vi "启动.vi"() -> ()   [LabVIEW 2016]
uses:
  <vilib>/NI/Progress Bar/Controls/Update Bar Actions.ctl
  <vilib>/NI/Progress Bar/Controls/Progress Bar Properties.ctl
  <vilib>/NI/Progress Bar/Progress Bar.lvlib
panel:
  out "exists?":bool
  out "error out":errorcluster
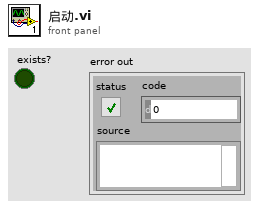
[diagram p1: front panel]
types:
  T1 = enum32{"Invalid", "Standard", "Closed", "Hidden", "Minimized", "Maximized"}
  T2 = typedef "Progress Bar.lvlib/Progress Bar Properties.ctl" = cluster{"Background Color":u32, "Installer Title":string, "Title Color":u32, "Action Text":string, "Text Color":u32, "Slider Value":u8, "Bar Color":u32, "Timeout":i32}
  T3 = typedef "Progress Bar.lvlib/Update Bar Actions.ctl" = enum16{"Add To Existing", "Set to Value"}
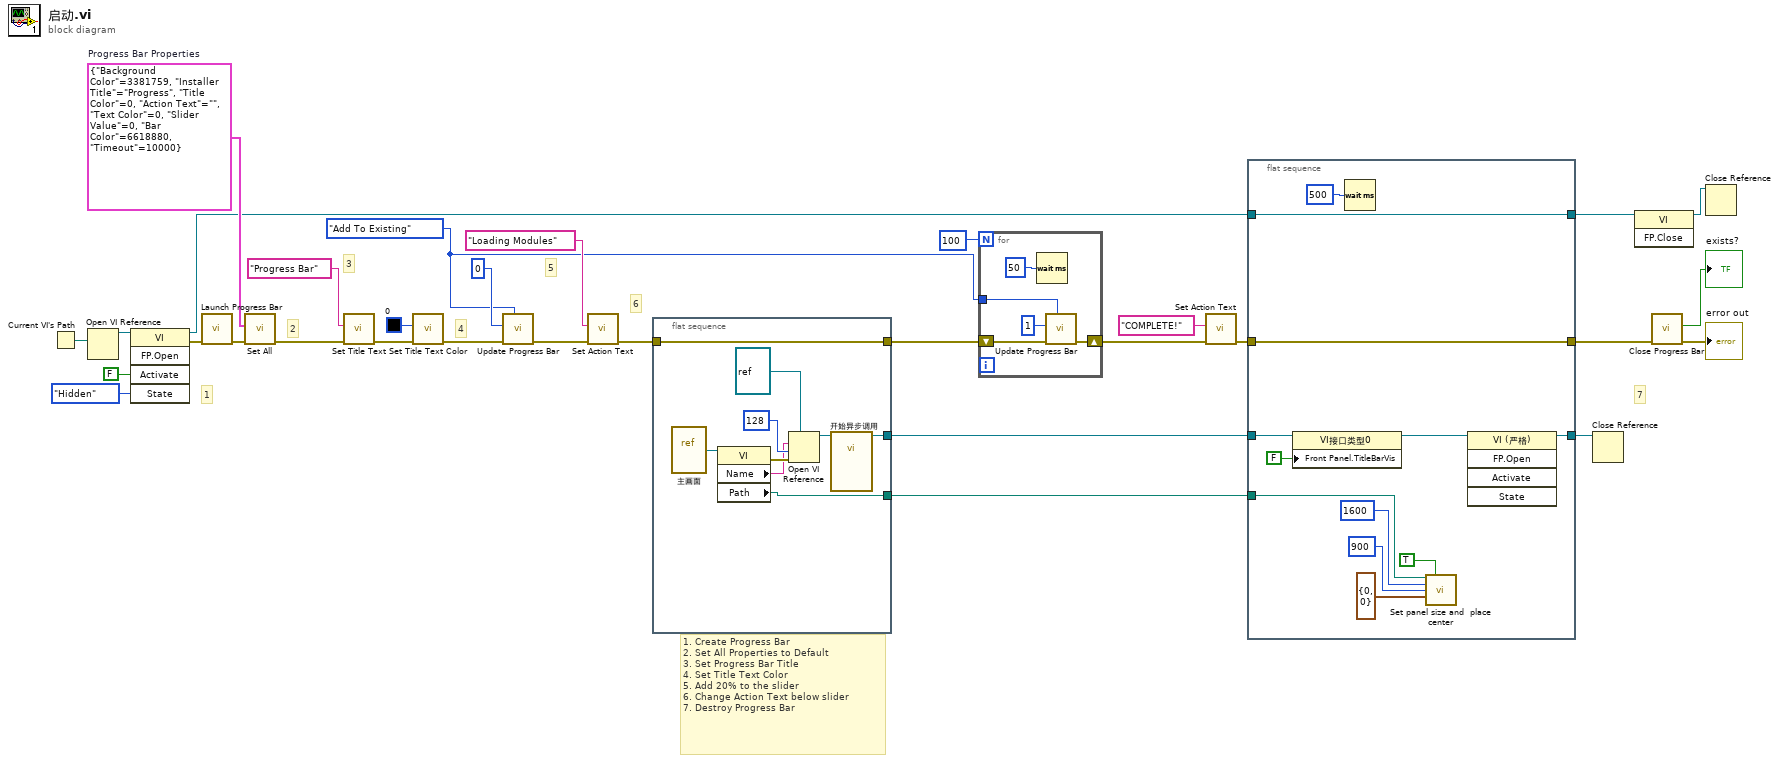
[diagram p0: block diagram]
diagram:
  w16 = T2 {"Background Color"=3381759, "Installer Title"="Progress", "Title Color"=0, "Action Text"="", "Text Color"=0, "Slider Value"=0, "Bar Color"=6618880, "Timeout"=10000}  # Progress Bar Properties
  w15 = Update_Bar_Actions."Add To Existing" ("Action")
  # "7"
  # "6"
  # "5"
  # "4"
  # "3"
  # "2"
  # "1"
  # "1. Create Progress Bar\n2. Set All Properties to Default\n3. Set Progress Bar Title\n4. Set Title Text Color\n5. Add 20% to the slider\n6. Change Action Text below slider\n7. Destroy Progress Bar"
  n1 = Current VI's Path() -> (path=w5:path)
  n2 = Open VI Reference(vi path=w5) -> (vi reference=w6:refnum<vi>)  [unwired: 5 in, 1 out]
  n3 = invoke class="VI" method="FP.Open"(reference=w6, "Activate"=FALSE ("激活？"), "State"=T1."Hidden" ("状态")) -> (reference out=w1:refnum<vi>, error out=w2:errorcluster)  [unwired: 2 in, 3 out]
  n4 = call <vilib>:"Launch Progress Bar.vi"("error in (no error)"=w2) -> ("error out"=w17:errorcluster)  [unwired: 9 in, 1 out]
  n5 = call <vilib>:"Set All.vi"("error in (no error)"=w17, "Progress Bar Properties (Default)"=w16) -> ("error out"=w27:errorcluster)  [unwired: 9 in]
  n6 = call <vilib>:"Set Title Text.vi"("error in (no error)"=w27, "Installer Title"="Progress Bar") -> ("error out"=w30:errorcluster)  [unwired: 9 in]
  n7 = call <vilib>:"Set Title Text Color.vi"("error in (no error)"=w30, "Color Box"=u32 0) -> ("error out"=w26:errorcluster)  [unwired: 9 in]
  n8 = call <vilib>:"Update Progress Bar.vi"("Action"=w15, "error in (no error)"=w26, "Value"=u8 0) -> ("error out"=w25:errorcluster)  [unwired: 8 in]
  n9 = call <vilib>:"Set Action Text.vi"("error in (no error)"=w25, "Action Text"="Loading Modules") -> ("error out"=w24:errorcluster)  [unwired: 9 in]
  n10 = flat-sequence {
    tunnel: w24 -> [w40]
    tunnel: [w40] -> w22
    tunnel: [w39] -> w9
    tunnel: [w32] -> w7
    frame #0 {
      n11 = vi-ref "主画面.vi"() -> (w34:refnum<vi>)
      n12 = property class="VI"(reference=w34) -> (error out=w38:errorcluster, "Name"=w35:string, "Path"=w32:path)  [unwired: 1 in, 1 out]
      n13 = Open VI Reference(type specifier VI Refnum (for type only)=refnum<vi> refnum ("类型说明符VI引用句柄（仅用于类型）"), vi path=w35, options=128 ("选项"), error in (no error)=w38) -> (vi reference=w33:refnum<vi>)  [unwired: 2 in, 1 out]
      n14 = call-by-ref "开始异步调用"(reference=w33) -> (reference out=w39:refnum<vi>)  [unwired: 13 in, 1 out]
    }
  }
  n15 = for {
    N: 100 ("Value") -> [_]
    tunnel: w15 -> [w42]
    shift-right: [w45] -> w21
    shift-left: w22 -> [w44]
    n16 = Wait (ms)(milliseconds to wait=u32 50) -> ()  [unwired: 1 out]
    n17 = call <vilib>:"Update Progress Bar.vi"("Action"=w42, "error in (no error)"=w44, "Value"=u8 1) -> ("error out"=w45:errorcluster)  [unwired: 8 in]
  }
  n18 = call <vilib>:"Set Action Text.vi"("error in (no error)"=w21, "Action Text"="COMPLETE!") -> ("error out"=w20:errorcluster)  [unwired: 9 in]
  n19 = flat-sequence {
    tunnel: w20 -> [w56]
    tunnel: [w56] -> w18
    tunnel: [w55] -> w10
    tunnel: w1 -> [w55]
    tunnel: w9 -> [w48]
    tunnel: [w54] -> w8
    tunnel: w7 -> [w49]
    frame #0 {
      n20 = property class="VI接口类型0"(reference=w48, "Front Panel.TitleBarVis"=FALSE ("前面板窗口:标题栏可见")) -> (reference out=w47:refnum<vi>)  [unwired: 1 in, 1 out]
      n21 = Wait (ms)(milliseconds to wait=u32 500) -> ()  [unwired: 1 out]
      n22 = call "Set panel size and  place center.vi"("Path"=w49, "Close Reference (false)"=TRUE, "Panel Width"=1600, "Panel Height"=900, "FP.Origin in(H & V)"=cluster{"Horizontal":i16, "Vertical":i16} {"Horizontal"=0, "Vertical"=0}) -> ()  [unwired: 6 in, 5 out]
      n23 = invoke class="VI (严格)" method="FP.Open"(reference=w47) -> (reference out=w54:refnum<vi>)  [unwired: 4 in, 4 out]
    }
  }
  n24 = Close Reference(reference=w8) -> ()  [unwired: 1 in, 1 out]
  n25 = invoke class="VI" method="FP.Close"(reference=w10) -> (reference out=w11:refnum<vi>)  [unwired: 2 in, 2 out]
  n26 = call <vilib>:"Close Progress Bar.vi"("error in (no error)"=w18) -> ("error out"=→"error out":errorcluster, "exists?"=→"exists?":bool)  [unwired: 9 in]
  n27 = Close Reference(reference=w11) -> ()  [unwired: 1 in, 1 out]
